vi "Main_Var.vi"() -> (0 "Var":T3)   [LabVIEW 2015]
uses:
  <vilib>/Rock Robotics/WPI/DriverStation/WPI_DriverStationRobotMode2.ctl
  <vilib>/Rock Robotics/WPI/Camera/WPI_CameraImageSize.ctl
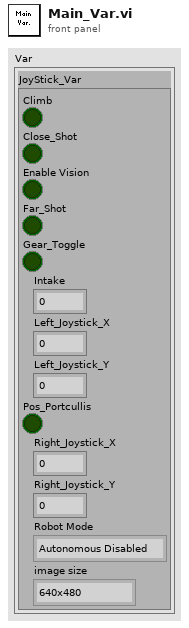
[diagram p1: front panel]
types:
  T1 = typedef "WPI_DriverStationRobotMode2.ctl" = enum16{"Autonomous Disabled", "Autonomous Enabled", "Teleop Disabled", "Teleop Enabled", "Disconnected", "Finish", "Test Disabled", "Test Enabled", "Emergency Stopped"}
  T2 = typedef "WPI_CameraImageSize.ctl" = enum16{"640x480", "320x240", "160x120", "Custom"}
  T3 = cluster{"JoyStick_Var":cluster{"Climb":bool, "Close_Shot":bool, "Enable Vision":bool, "Far_Shot":bool, "Gear_Toggle":bool, "Intake":dbl, "Left_Joystick_X":dbl, "Left_Joystick_Y":dbl, "Pos_Portcullis":bool, "Right_Joystick_X":dbl, "Right_Joystick_Y":dbl, "Robot Mode":T1, "image size":T2}}
  T4 = cluster{"Climb":bool, "Close_Shot":bool, "Enable Vision":bool, "Far_Shot":bool, "Gear_Toggle":bool, "Intake":dbl, "Left_Joystick_X":dbl, "Left_Joystick_Y":dbl, "Pos_Portcullis":bool, "Right_Joystick_X":dbl, "Right_Joystick_Y":dbl, "Robot Mode":T1, "image size":T2}
  T5 = cluster{"JoyStick":cluster{"Climb":bool, "Close_Shot":bool, "Enable Vision":bool, "Far_Shot":bool, "Gear_Toggle":bool, "Intake":dbl, "Left_Joystick_X":dbl, "Left_Joystick_Y":dbl, "Pos_Portcullis":bool, "Right_Joystick_X":dbl, "Right_Joystick_Y":dbl, "Robot Mode":T1, "image size":T2}}
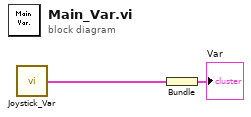
[diagram p0: block diagram]
diagram:
  n1 = call "Joystick_Var.vi"() -> ("JoyStick"=w2:T4)
  n2 = Bundle("JoyStick"=w2) -> (→"Var":T5)  [unwired: 1 in]
